vi "Normalise.vi"(11 "Vector 2D in":refnum<class "Vector 2D.lvclass">) -> (3 "Vector 2D out":refnum<class "Vector 2D.lvclass">)   [LabVIEW 2021, in "Vector 2D.lvclass"]
uses:
  Vector 2D.lvclass
  Vector 2D.lvclass/Vector 2D.ctl
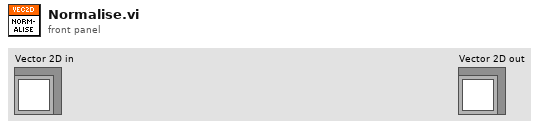
[diagram p1: front panel]
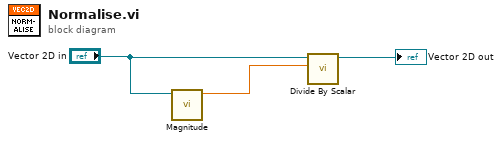
[diagram p0: block diagram]
diagram:
  n1 = call "Magnitude.vi"("A"="Vector 2D in") -> ("Magnitude"=w2:sgl)  [unwired: 10 in]
  n2 = call "Divide By Scalar.vi"("x"=w2, "A"="Vector 2D in") -> ("Ax"=→"Vector 2D out":refnum<class "Vector 2D.lvclass">)  [unwired: 9 in]
